vi "TSPopup.Demo tree Registration.vi"(0 "TSPopup in":refnum<class "TSPopup.lvclass">, 1 "Signal Settings ref":refnum<vi>, 3 "error in (no error)":errorcluster) -> (6 "TSPopup out":refnum<class "TSPopup.lvclass">, 7 "dup ref out":refnum<vi>, 9 "error out":errorcluster)   [LabVIEW 2016, in "TSPopup.lvlib" / "TSPopup.lvclass"]
doc: "VI to hold all the different type registrations for this specific demo.\n\nType Sensitive Popup \nCopyright © 2007, J. David Saunders\nAll rights reserved."
uses:
  <userlib>/TSPopup/TSPopup.lvclass
  <userlib>/TSPopup/TSPopup.Popup Call Parameters.ctl
  <userlib>/TSPopup/TSPopup.Data Type.ctl
panel:
  in  "Show Popup (type only)":T1
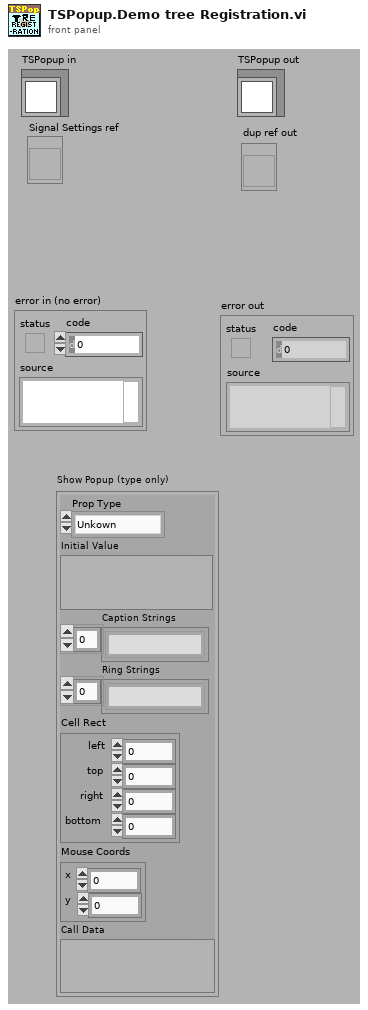
[diagram p1: front panel]
types:
  T1 = typedef "TSPopup.lvlib/TSPopup.lvclass/TSPopup.Popup Call Parameters.ctl" = cluster{"Prop Type":T2, "Initial Value":variant, "Caption Strings":string[], "Ring Strings":string[], "Cell Rect":cluster{"left":i16, "top":i16, "right":i16, "bottom":i16}, "Mouse Coords":cluster{"x":i16, "y":i16}, "Call Data":variant}
  T2 = typedef "TSPopup.lvlib/TSPopup.lvclass/TSPopup.Data Type.ctl" = enum16{"Unkown", "NO POPUP", "String", "Integer", "Float", "Color", "Boolean", "Ring", "Captioned String", "Captioned Integer", "Button Color", "2 Int Cluster", "4 Int Cluster", "check"}
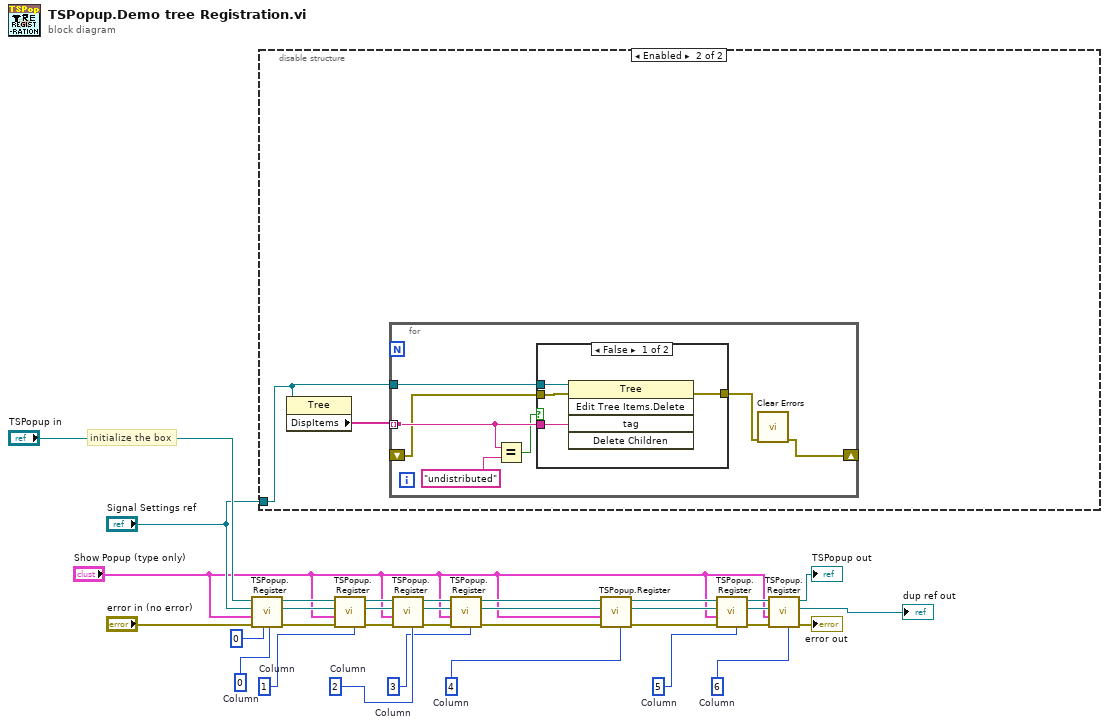
[diagram p0: block diagram]
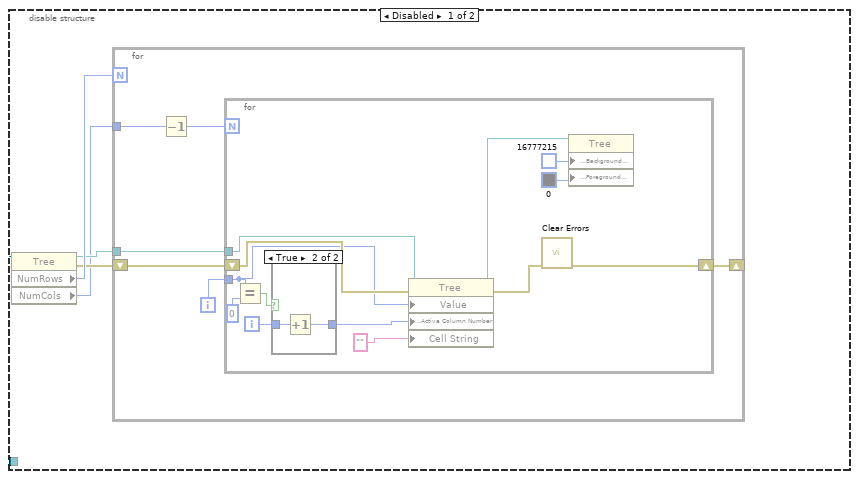
[diagram p2: hidden frame]
diagram:
  w5 = 6  # Column
  w31 = 0  # Column
  w11 = 5  # Column
  w16 = 4  # Column
  w24 = 2  # Column
  w27 = 1  # Column
  w19 = 3  # Column
  # "initialize the box"
  n1 = call <userlib>:"TSPopup.Register.vi"("Col (unwired = all columns)"=w31, "Row (unwired = all rows)"=0, "error in (no error)"="error in (no error)", "Parameters"="Show Popup (type only)", "Ctl Refnum"="Signal Settings ref", "TSPopup in"="TSPopup in") -> ("error out"=w28:errorcluster, "dup ref out"=w29:refnum<vi>, "TSPopup out"=w30:refnum<class "TSPopup.lvclass">)  [unwired: 3 in]
  n2 = disable-structure shown="Enabled" {
    disable-tunnel: "Signal Settings ref" -> [w38 w61]
    frame Disabled {
      n3 = property class="Tree"(reference=w38) -> (reference out=w36:refnum<vi>, error out=w35:errorcluster, "NumRows"=w37:u32, "NumCols"=w34:u32)  [unwired: 1 in]
      n4 = for {
        N: w37 -> [_]
        tunnel: w36 -> [w44]
        shift-right: [w41] -> _
        shift-left: w35 -> [w42]
        tunnel: w34 -> [w40]
        i -> [w43]
        n5 = Decrement(x=w40) -> (x-1=w39:u32)
        n6 = for {
          N: w39 -> [_]
          tunnel: w44 -> [w57]
          tunnel: w43 -> [w45]
          shift-right: [w50] -> w41
          shift-left: w42 -> [w52]
          i -> [w49]
          n7 = Equal?(x=w45, y=0) -> (x = y?=w46:bool)
          n8 = case shown="True" w46 {
            tunnel: w49 -> [w58 w60]
            tunnel: [w58 w59] -> w48
            frame False {
            }
            frame True {
              n9 = Increment(x=w60) -> (x+1=w59:i32)
            }
          }
          n10 = property class="Tree"(reference=w57, error in=w52, "Value"=w45, "Active Cell:Active Column Number"=w48, "Cell String"="" ("Active Cell:String")) -> (reference out=w54:refnum<vi>, error out=w51:errorcluster)
          n11 = call <vilib>:"Clear Errors.vi"("error in (no error)"=w51) -> ("error out"=w50:errorcluster)  [unwired: 5 in, 1 out]
          n12 = property class="Tree"(reference=w54, "Active Cell:Background Color"=u32 16777215, "Active Cell:Foreground Color"=u32 0) -> ()  [unwired: 1 in, 2 out]
        }
      }
    }
    frame Enabled {
      n13 = property class="Tree"(reference=w61) -> ("DispItems"=w62:string[])  [unwired: 1 in, 2 out]
      n14 = for {
        tunnel: w62 -> [w68] mode=indexing
        tunnel: w61 -> [w69]
        shift-right: [w64] -> _
        shift-left: _ -> [w63]
        n15 = Equal?(x=w68, y="undistributed") -> (x = y?=w66:bool)
        n16 = case shown="False" w66 {
          tunnel: w69 -> [w73 _]
          tunnel: w68 -> [w72 _]
          tunnel: [w71 w74] -> w65
          tunnel: w63 -> [w70 w74]
          frame False {
            n17 = invoke on="Invoke Node" class="Tree" method="Edit Tree Items.Delete"(reference=w73, error in=w70, "tag"=w72) -> (error out=w71:errorcluster)  [unwired: 2 in, 4 out]
          }
          frame True {
          }
        }
        n18 = call <vilib>:"Clear Errors.vi"("error in (no error)"=w65) -> ("error out"=w64:errorcluster)  [unwired: 5 in, 1 out]
      }
    }
  }
  n19 = call <userlib>:"TSPopup.Register.vi"("Col (unwired = all columns)"=w27, "error in (no error)"=w28, "Parameters"="Show Popup (type only)", "Ctl Refnum"=w29, "TSPopup in"=w30) -> ("error out"=w20:errorcluster, "dup ref out"=w25:refnum<vi>, "TSPopup out"=w26:refnum<class "TSPopup.lvclass">)  [unwired: 4 in]
  n20 = call <userlib>:"TSPopup.Register.vi"("Col (unwired = all columns)"=w24, "error in (no error)"=w20, "Parameters"="Show Popup (type only)", "Ctl Refnum"=w25, "TSPopup in"=w26) -> ("error out"=w21:errorcluster, "dup ref out"=w22:refnum<vi>, "TSPopup out"=w23:refnum<class "TSPopup.lvclass">)  [unwired: 4 in]
  n21 = call <userlib>:"TSPopup.Register.vi"("Col (unwired = all columns)"=w19, "error in (no error)"=w21, "Parameters"="Show Popup (type only)", "Ctl Refnum"=w22, "TSPopup in"=w23) -> ("error out"=w12:errorcluster, "dup ref out"=w17:refnum<vi>, "TSPopup out"=w18:refnum<class "TSPopup.lvclass">)  [unwired: 4 in]
  n22 = call <userlib>:"TSPopup.Register.vi"("Col (unwired = all columns)"=w16, "error in (no error)"=w12, "Parameters"="Show Popup (type only)", "Ctl Refnum"=w17, "TSPopup in"=w18) -> ("error out"=w13:errorcluster, "dup ref out"=w14:refnum<vi>, "TSPopup out"=w15:refnum<class "TSPopup.lvclass">)  [unwired: 4 in]
  n23 = call <userlib>:"TSPopup.Register.vi"("Col (unwired = all columns)"=w11, "error in (no error)"=w13, "Parameters"="Show Popup (type only)", "Ctl Refnum"=w14, "TSPopup in"=w15) -> ("error out"=w7:errorcluster, "dup ref out"=w9:refnum<vi>, "TSPopup out"=w10:refnum<class "TSPopup.lvclass">)  [unwired: 4 in]
  n24 = call <userlib>:"TSPopup.Register.vi"("Col (unwired = all columns)"=w5, "error in (no error)"=w7, "Parameters"="Show Popup (type only)", "Ctl Refnum"=w9, "TSPopup in"=w10) -> ("error out"=→"error out":errorcluster, "dup ref out"=→"dup ref out":refnum<vi>, "TSPopup out"=→"TSPopup out":refnum<class "TSPopup.lvclass">)  [unwired: 4 in]
